vi "temseq_new.vi"() -> ()   [LabVIEW 2015]
uses:
  BERTTA.dll
panel:
  out "0, 1":i16
  out "Waveform Chart":dynamicdata(graph)
  in  "port":i32=9
  out "elapsed":i32
  out "params":dbl[](array[numeric])
  in  "TimeParams":i32[](array[numeric])=[6, 5, 5, 5, 5]
  in  "SeqParams":dbl[](array[numeric])=[20.0, 35.0, 45.0, 20.0, 20.0, 35.0, 45.0, 20.0, 20.0, 20.0, 20.0, 20.0, 20.0, 20.0, 20.0, 40.0, 2.5, 1.0]
  out "Tr":dbl
  in  "Tr_orTj":i32
  in  "shutdown":i32
  in  "pause":i32
  in  "master":i32
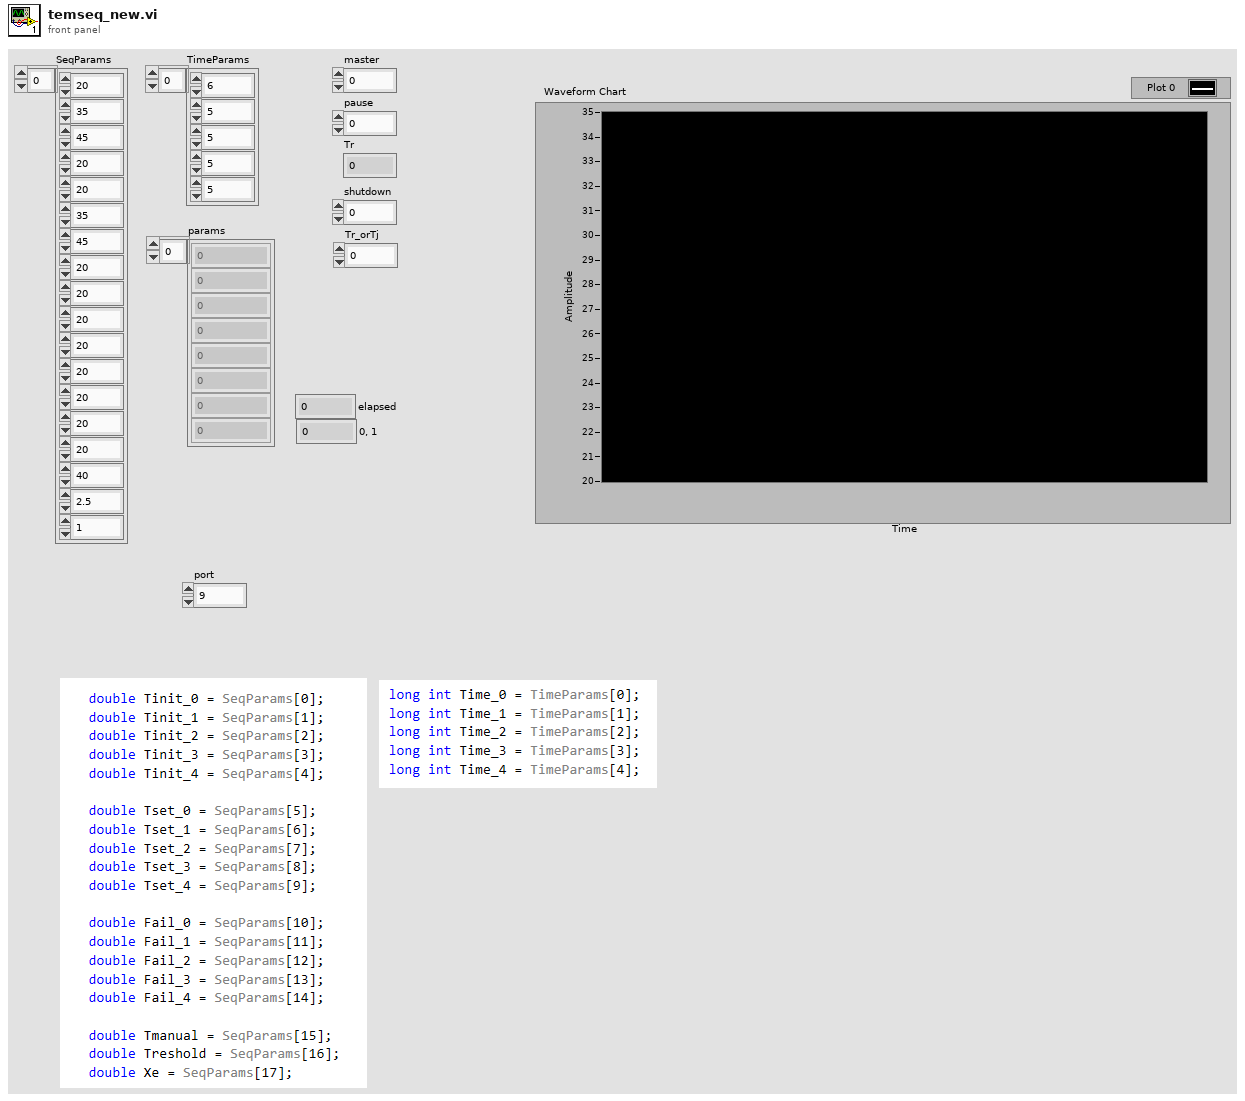
[diagram p1: front panel]
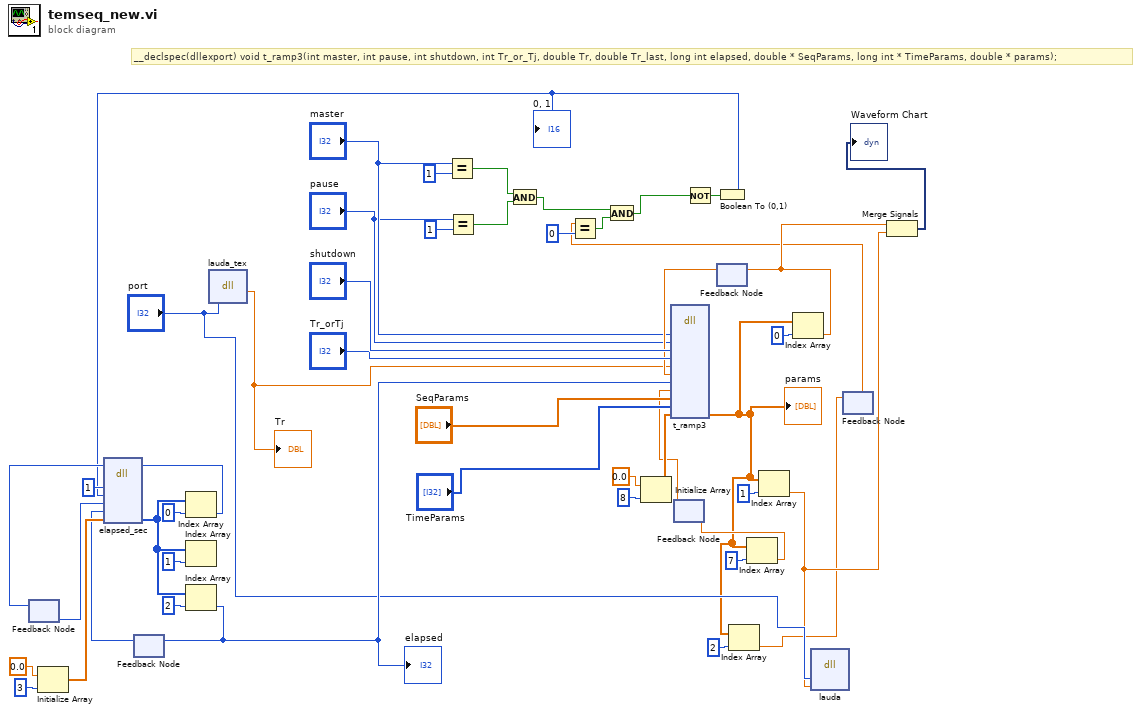
[diagram p0: block diagram]
diagram:
  # "__declspec(dllexport) void t_ramp3(int master, int pause, int shutdown, int Tr_or_Tj, double Tr, double Tr_last, long int elapsed, double * SeqParams, long int * TimeParams, double * params);"
  n1 = feedback #1() -> (w29:i32)  [unwired: 1 in]
  n2 = Initialize Array(0.0 ("element"), 3 ("dimension size")) -> (w34:dbl[])
  n3 = feedback #2() -> (w28:i32)  [unwired: 1 in]
  n4 = dll-call lib="C:/Users/shresplab/OneDrive - Kemira Oyj/Documents/Visual Studio 2017/Projects/Bertta/BERTTA/x64/Debug/BERTTA.dll" fn="lauda_tex"("port"="port") -> ("return type"=w15:dbl)  [unwired: 4 in, 2 out]
  "Tr" <- w15
  n5 = Equal?(x="master", y=1) -> (x = y?=w21:bool)
  n6 = Equal?(x="pause", y=1) -> (x = y?=w20:bool)
  n7 = And(x=w21, y=w20) -> (x .and. y?=w7:bool)
  n8 = Initialize Array(0.0 ("element"), 8 ("dimension size")) -> (w40:dbl[])
  n9 = feedback #3() -> (w9:dbl)  [unwired: 1 in]
  n10 = feedback #4() -> (w38:dbl)  [unwired: 1 in]
  n11 = feedback #5() -> (w1:dbl)  [unwired: 1 in]
  n12 = Equal?(x=w1, y=0) -> (x = y?=w5:bool)
  n13 = And(x=w7, y=w5) -> (x .and. y?=w6:bool)
  n14 = Not(x=w6) -> (.not. x?=w19:bool)
  n15 = Boolean To (0,1)(Boolean=w19) -> (0, 1=w18:i16)
  "0, 1" <- w18
  n16 = dll-call lib="C:/Users/shresplab/OneDrive - Kemira Oyj/Documents/Visual Studio 2017/Projects/Bertta/BERTTA/x64/Debug/BERTTA.dll" fn="elapsed_sec"("enable"=1, "reset"=w18, "last_time"=w29, "elapsed_last"=w28, "params"=w34) -> ("params"=w31:i32[])  [unwired: 8 in, 2 out]
  n17 = Index Array(array=w31, index=0) -> (element=w30:i32)
  n18 = feedback-in #1(w30) -> ()
  n19 = Index Array(array=w31, index=1) -> ()  [unwired: 1 out]
  n20 = Index Array(array=w31, index=2) -> (element=w27:i32)
  "elapsed" <- w27
  n21 = feedback-in #2(w27) -> ()
  n22 = dll-call lib="C:/Users/shresplab/OneDrive - Kemira Oyj/Documents/Visual Studio 2017/Projects/Bertta/BERTTA/x64/Debug/BERTTA.dll" fn="t_ramp3"("master"="master", "pause"="pause", "shutdown"="shutdown", "Tr_orTj"="Tr_orTj", "Tr"=w15, "Tr_last"=w38, "elapsed"=w27, "step_previous"=w9, "SeqParams"="SeqParams", "TimeParams"="TimeParams", "params"=w40) -> ("params"=w3:dbl[])  [unwired: 14 in, 2 out]
  "params" <- w3
  n23 = Index Array(array=w3, index=2) -> (element=w2:dbl)
  n24 = Index Array(array=w3, index=7) -> (element=w10:dbl)
  n25 = feedback-in #3(w10) -> ()
  n26 = Index Array(array=w3, index=1) -> (element=w13:dbl)
  n27 = Index Array(array=w3, index=0) -> (element=w14:dbl)
  n28 = feedback-in #4(w14) -> ()
  n29 = dll-call lib="C:/Users/shresplab/OneDrive - Kemira Oyj/Documents/Visual Studio 2017/Projects/Bertta/BERTTA/x64/Debug/BERTTA.dll" fn="lauda"("port"="port", "set_temp"=w13) -> ()  [unwired: 6 in, 2 out]
  n30 = feedback-in #5(w2) -> ()
  n31 = Merge Signals(w14, w13) -> (→"Waveform Chart":dynamicdata)
